vi "gradient_ascent_2d.vi"() -> ()   [LabVIEW 2024]
uses:
  O:/DSG/Tyler/EIC/DIRC/daq/automated/Thorlabs.MotionControl.IntegratedStepperMotorsCLI.dll
  Thorlabs.MotionControl.IntegratedStepperMotorsCLI.dll
panel:
  in  "pdx_dev":refnum<k24>
  in  "pdy_dev":refnum<k24>
  in  "z_in":dbl
  in  "pos_in":dbl[](array[numeric])=[75.0, 72.0]
  in  "N trials":dbl=16.0
  out "end result":dbl[](array[numeric])
  in  "k":dbl=25.0
  # "Used only to create Gaussian to optimize"
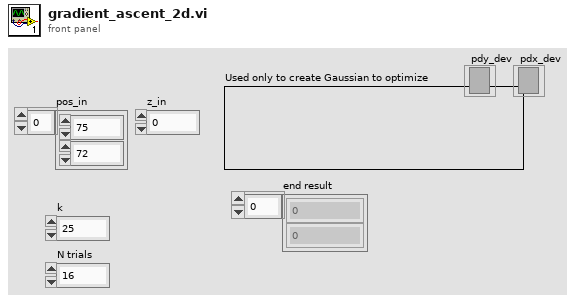
[diagram p1: front panel]
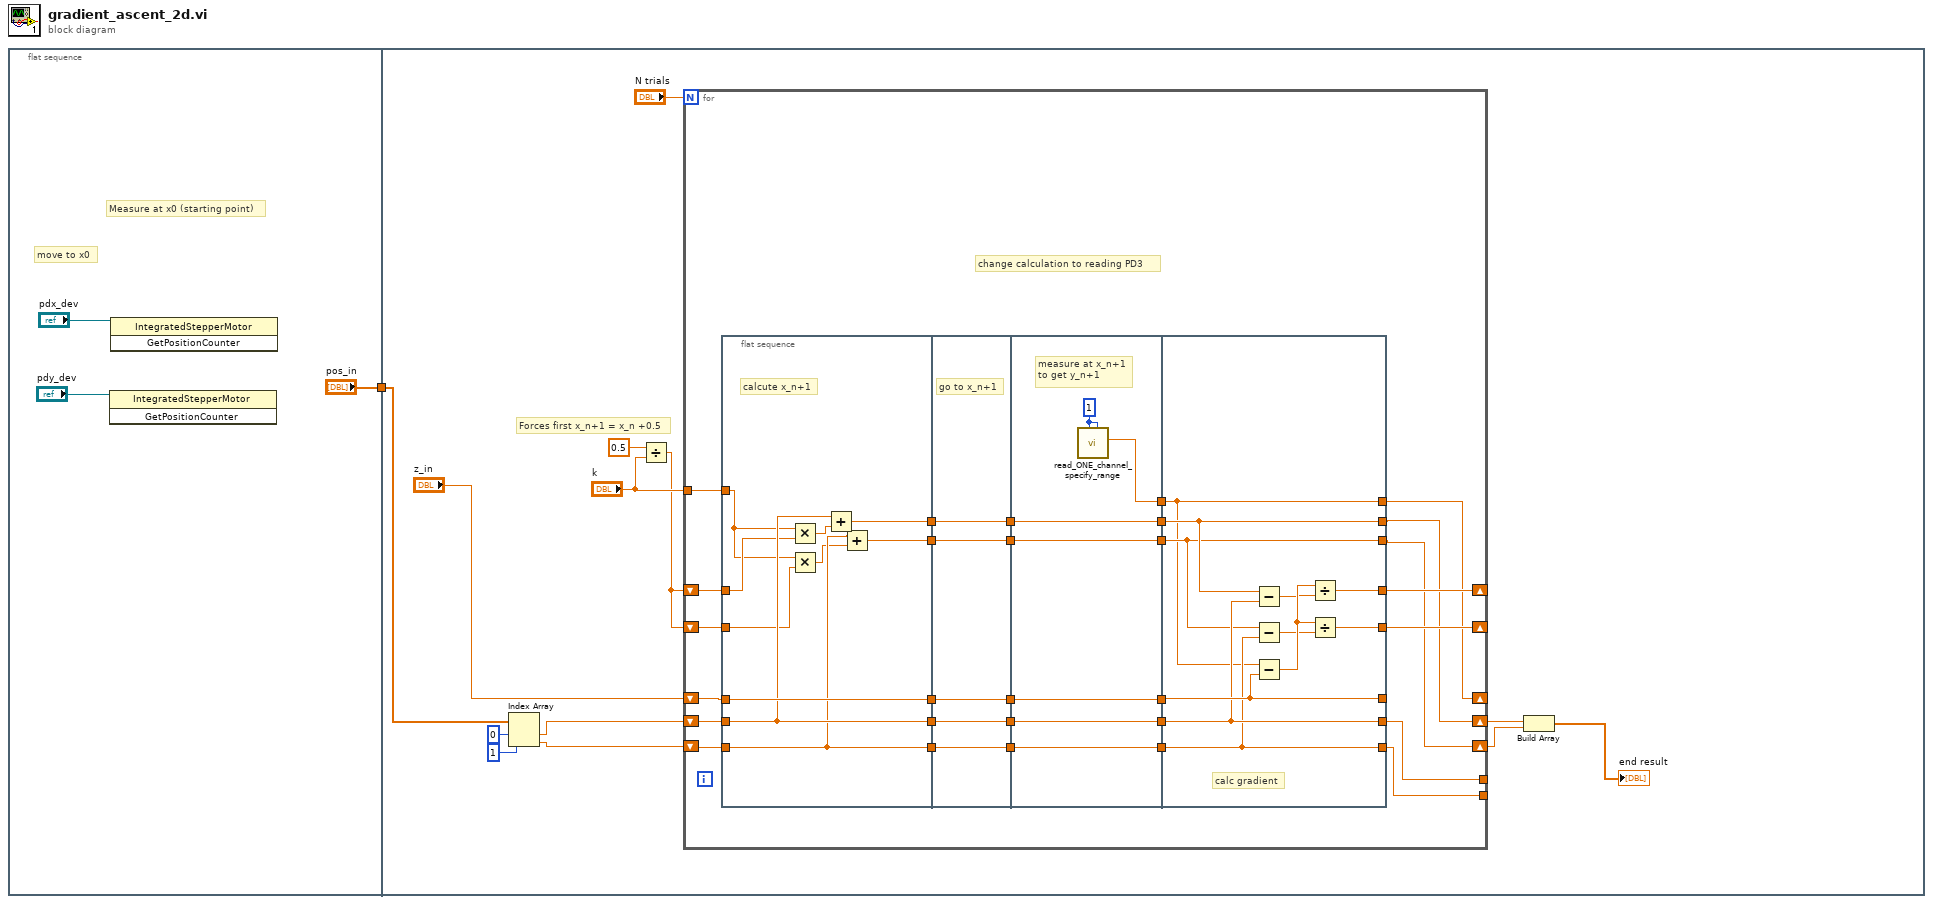
[diagram p0: block diagram]
diagram:
  n1 = flat-sequence {
    tunnel: ["pos_in"] -> w1
    tunnel: w1 -> [w17]
    frame #0 {
      # "move to x0"
      # "Measure at x0 (starting point)"
      n2 = invoke class="IntegratedStepperMotor" method="GetPositionCounter"(reference="pdy_dev") -> ()  [unwired: 2 in, 3 out]
      n3 = invoke class="IntegratedStepperMotor" method="GetPositionCounter"(reference="pdx_dev") -> ()  [unwired: 2 in, 3 out]
    }
    frame #1 {
      # "Forces first x_n+1 = x_n +0.5"
      n4 = Index Array(array=w17, index #1=0 ("index"), index #2=1 ("index")) -> (element #1=w11:dbl, element #2=w10:dbl)
      n5 = Divide(x=0.5, y="k") -> (x/y=w9:dbl)
      n6 = for {
        N: "N trials" -> [_]
        shift-right: [w21] -> w7
        shift-left: w11 -> [w38]
        shift-right: [w22] -> _
        shift-left: "z_in" -> [w39]
        tunnel: "k" -> [w46]
        shift-right: [w20] -> w6
        shift-left: w10 -> [w32]
        shift-right: [w25] -> _
        shift-left: w9 -> [w23]
        shift-right: [w26] -> _
        shift-left: w9 -> [w24]
        tunnel: [w19] -> _
        tunnel: [w18] -> _
        # "change calculation to reading PD3"
        n7 = flat-sequence {
          tunnel: w46 -> [w47]
          tunnel: [w56] -> w45
          tunnel: w39 -> [w55]
          tunnel: [w55] -> w42
          tunnel: w38 -> [w54]
          tunnel: [w54] -> w36
          tunnel: [w53] -> w33
          tunnel: w32 -> [w53]
          tunnel: [w51] -> w30
          tunnel: w24 -> [w50]
          tunnel: w23 -> [w48]
          tunnel: w45 -> [w61]
          tunnel: [w61] -> w44
          tunnel: w42 -> [w60]
          tunnel: [w60] -> w41
          tunnel: [w59] -> w37
          tunnel: w36 -> [w59]
          tunnel: [w58] -> w34
          tunnel: w33 -> [w58]
          tunnel: w30 -> [w57]
          tunnel: [w57] -> w29
          tunnel: w44 -> [w65]
          tunnel: [w65] -> w43
          tunnel: w41 -> [w68]
          tunnel: [w68] -> w40
          tunnel: w37 -> [w67]
          tunnel: [w67] -> w35
          tunnel: w34 -> [w66]
          tunnel: [w66] -> w31
          tunnel: w29 -> [w64]
          tunnel: [w64] -> w28
          tunnel: [w63] -> w27
          tunnel: w43 -> [w74]
          tunnel: w40 -> [w79]
          tunnel: w35 -> [w78]
          tunnel: w31 -> [w77]
          tunnel: [w74] -> w21
          tunnel: w28 -> [w73]
          tunnel: [w73] -> w20
          tunnel: w27 -> [w69]
          tunnel: [w69] -> w22
          tunnel: [w79] -> _
          tunnel: [w78] -> w19
          tunnel: [w77] -> w18
          tunnel: [w76] -> w26
          tunnel: [w75] -> w25
          frame #0 {
            # "calcute x_n+1"
            n8 = Multiply(x=w47, y=w50) -> (x*y=w52:dbl)
            n9 = Multiply(x=w47, y=w48) -> (x*y=w49:dbl)
            n10 = Add(x=w54, y=w52) -> (x+y=w56:dbl)
            n11 = Add(x=w53, y=w49) -> (x+y=w51:dbl)
          }
          frame #1 {
            # "go to x_n+1"
          }
          frame #2 {
            w62 = u32 1 ("preDAQ  wait ms")
            # "measure at x_n+1\nto get y_n+1"
            n12 = call "read_ONE_channel_specify_range.vi"("postDAQ  wait ms"=w62, "preDAQ  wait ms"=w62) -> ("data"=w63:dbl)  [unwired: 7 in, 2 out]
          }
          frame #3 {
            # "calc gradient"
            n13 = Subtract(x=w74, y=w78) -> (x-y=w70:dbl)
            n14 = Subtract(x=w73, y=w77) -> (x-y=w71:dbl)
            n15 = Subtract(x=w69, y=w79) -> (x-y=w72:dbl)
            n16 = Divide(x=w72, y=w70) -> (x/y=w76:dbl)
            n17 = Divide(x=w72, y=w71) -> (x/y=w75:dbl)
          }
        }
      }
      n18 = Build Array(w7, w6) -> (→"end result":dbl[])
    }
  }
